vi "Get Message.vi"(8 "error in (no error)":errorcluster caption="entrée d'erreur (pas d'erreur)", 10 "Message type":T1="Control", 11 "GeneralFunctionality en entrée":refnum<class "GeneralFunctionality.lvclass">) -> (0 "error out":errorcluster caption="sortie d'erreur", 2 "Message.lvclass":refnum<class "Message.lvclass">, 3 "GeneralFunctionality en sortie":refnum<class "GeneralFunctionality.lvclass">)   [LabVIEW 2018, in "GeneralFunctionality.lvclass"]
uses:
  GeneralFunctionality.lvclass
  Message/Message.lvclass
  dependecies/ControlsVIs/Clusters-def/Message types.ctl
  GeneralFunctionality.lvclass/GeneralFunctionality.ctl
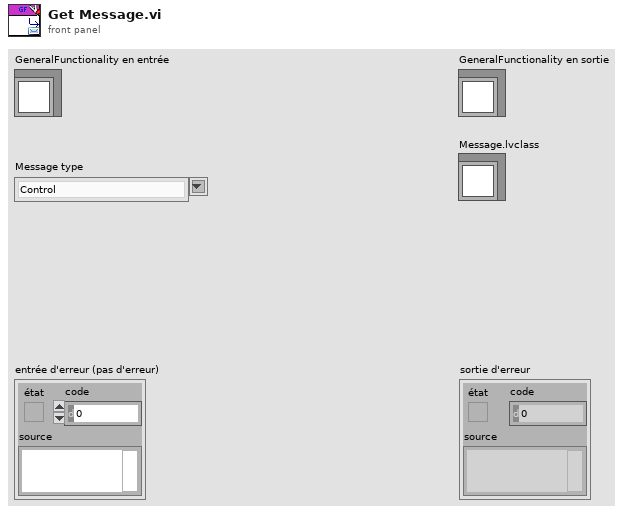
[diagram p1: front panel]
types:
  T1 = typedef "Message types.ctl" = string
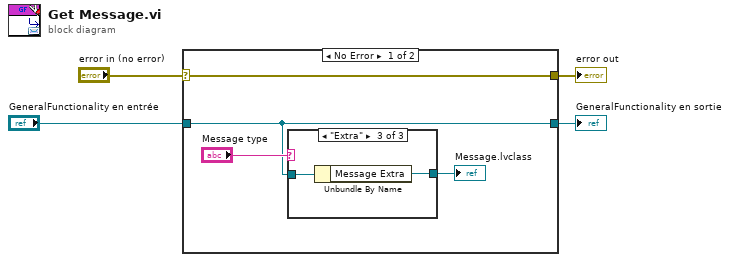
[diagram p0: block diagram]
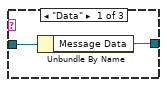
[diagram p2: hidden frame]
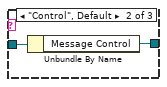
[diagram p3: hidden frame]
diagram:
  n1 = case shown="No Error" "error in (no error)" {
    selector: "error in (no error)" -> [w8 w16]
    tunnel: [w8 w16] -> w3
    tunnel: [w6 w15] -> w1
    tunnel: "GeneralFunctionality en entrée" -> [w6 w15]
    frame No Error {
      n2 = case shown="\"Extra\"" "Message type" {
        tunnel: w6 -> [w10 w12 w14]
        tunnel: [w9 w11 w13] -> w5
        frame "Data" {
          n3 = Unbundle By Name(w10) -> ("Message Data"=w9:refnum<class "Message.lvclass">)
        }
        frame "Control", Default {
          n4 = Unbundle By Name(w12) -> ("Message Control"=w11:refnum<class "Message.lvclass">)
        }
        frame "Extra" {
          n5 = Unbundle By Name(w14) -> ("Message Extra"=w13:refnum<class "Message.lvclass">)
        }
      }
      "Message.lvclass" <- w5
    }
    frame Error {
    }
  }
  "error out" <- w3
  "GeneralFunctionality en sortie" <- w1
